vi "Aero_tunnel_monitor.vi"() -> ()   [LabVIEW 2010]
panel:
  out "ROAD SPEED_mps":dbl
  in  "BL Fan1":i32
  in  "BL Fan2":i32
  in  "Stop drive":bool
  in  "Start Drive":bool
  in  "Synch to Wind":bool
  out "Road Info":string
  in  "stop":bool
  out "Lift":dbl caption="N" format="%#.2f"
  out "Pitch":dbl caption="N.m" format="%#.2f"
  out "Drag":dbl caption="N" format="%#.2f"
  out "Side-Force":dbl caption="N" format="%#.2f"
  out "Yaw":dbl caption="N.m" format="%#.2f"
  out "Roll":dbl caption="N.m" format="%#.2f"
  out "SmAD Data":dbl[](array[numeric]) format="%.2f"
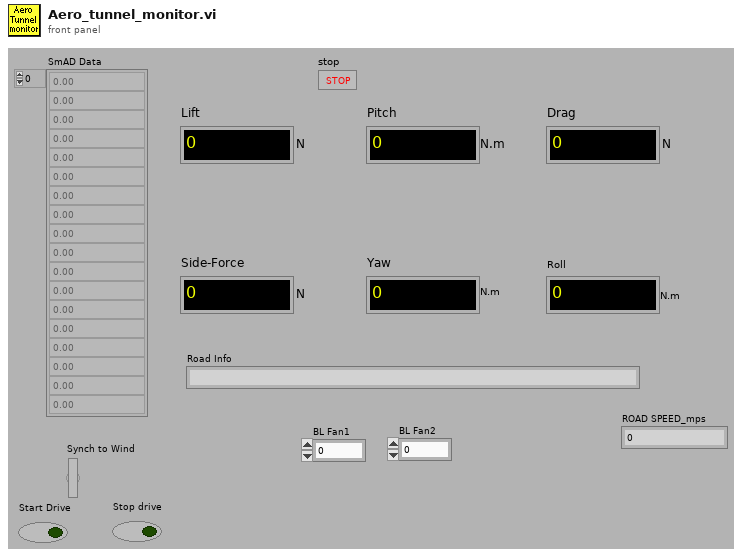
[diagram p1: front panel]
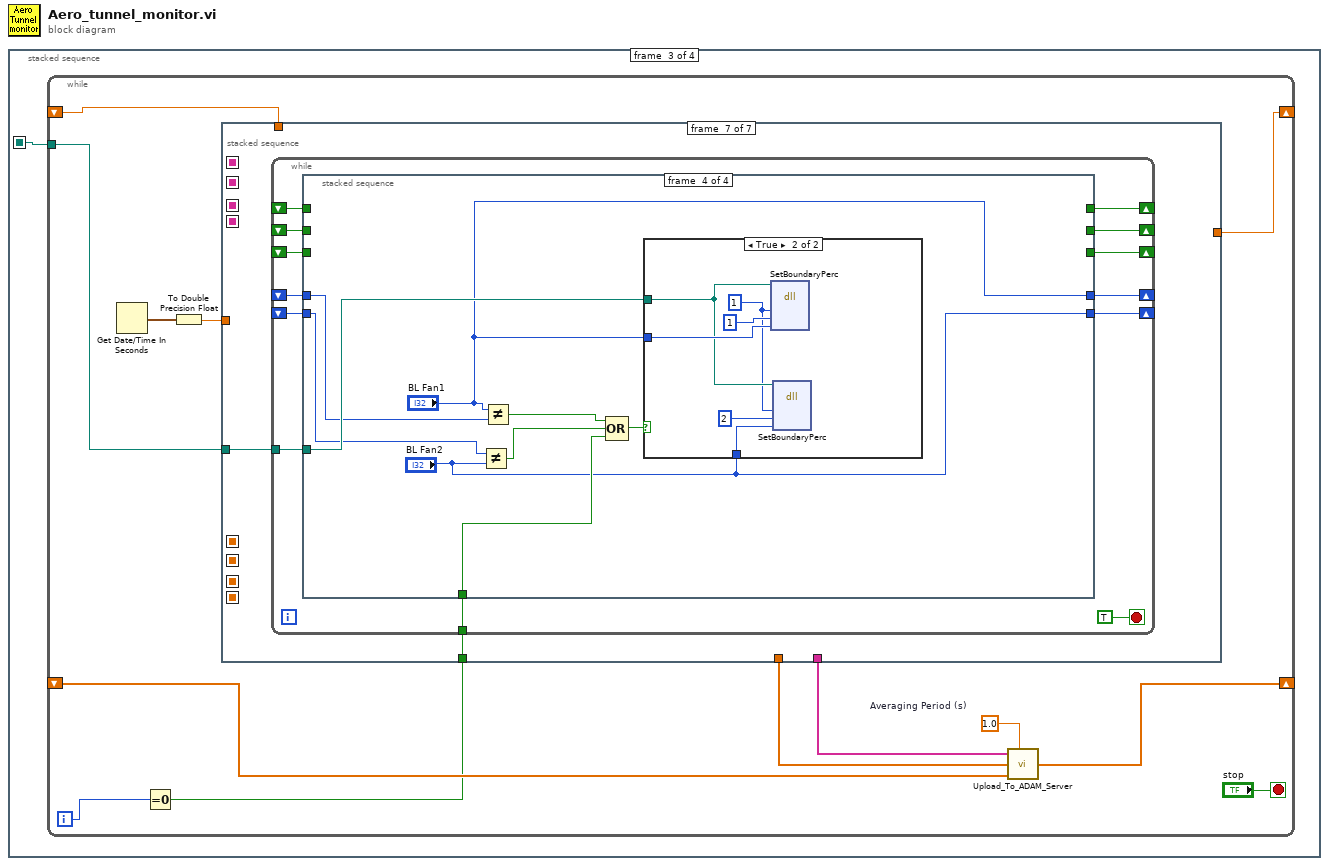
[diagram p0: block diagram]
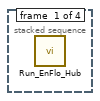
[diagram p2: hidden frame]
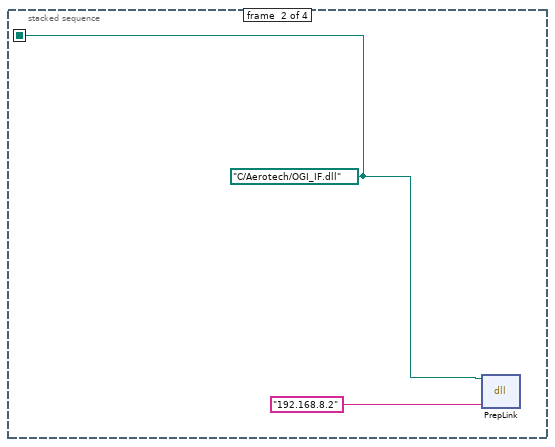
[diagram p3: hidden frame]
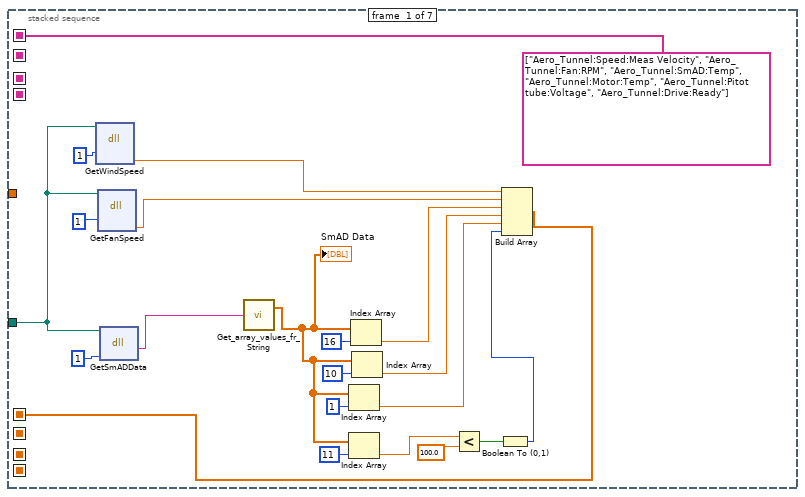
[diagram p4: hidden frame]
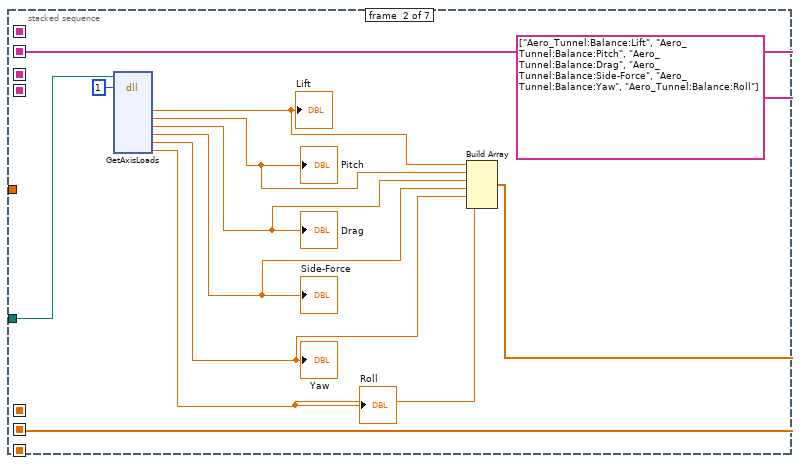
[diagram p5: hidden frame]
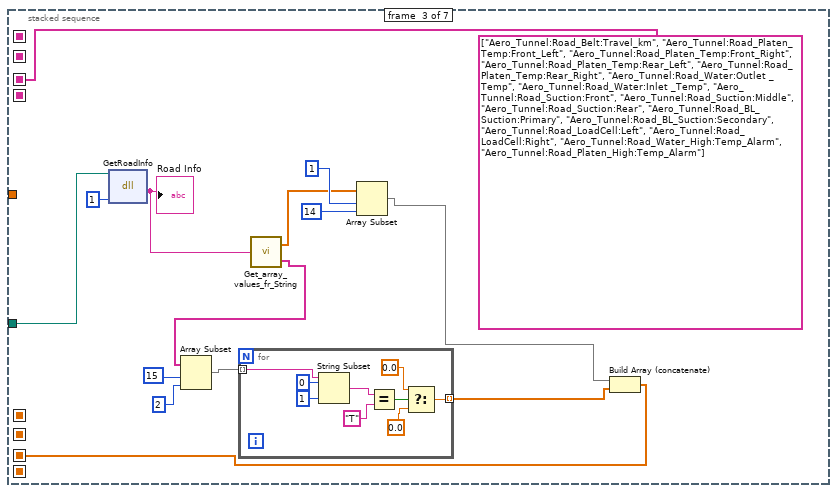
[diagram p6: hidden frame]
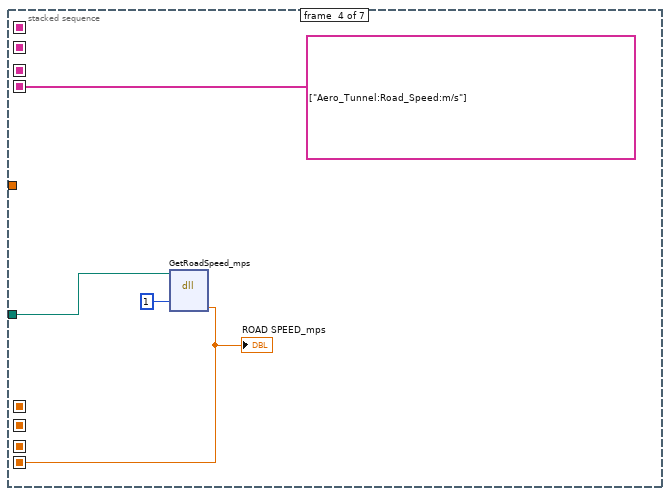
[diagram p7: hidden frame]
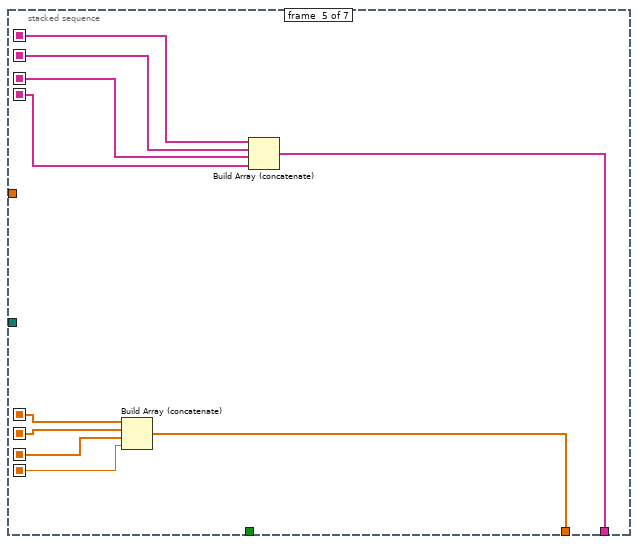
[diagram p8: hidden frame]
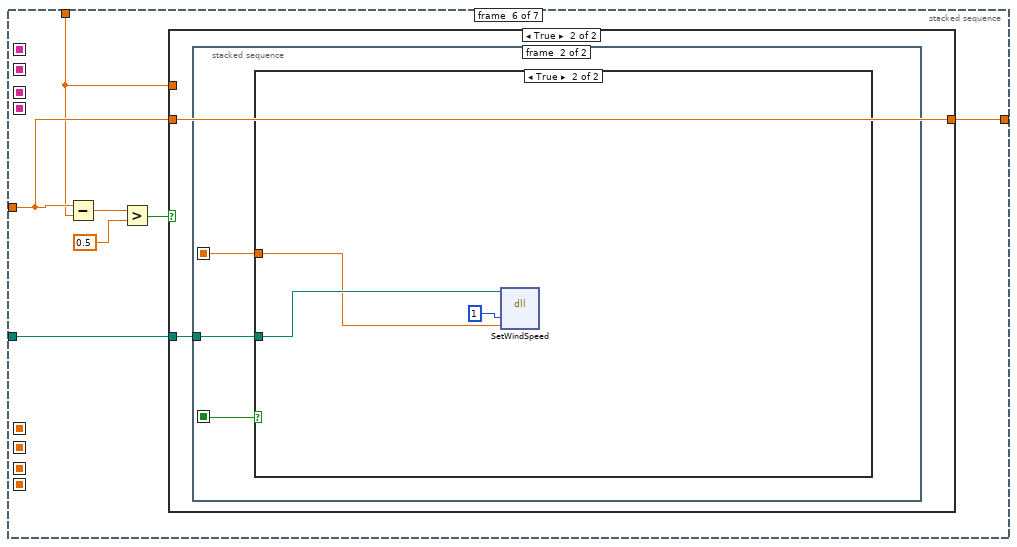
[diagram p9: hidden frame]
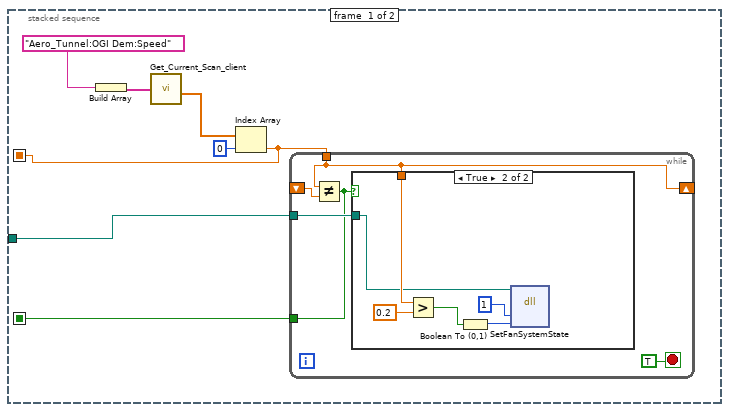
[diagram p11: hidden frame]
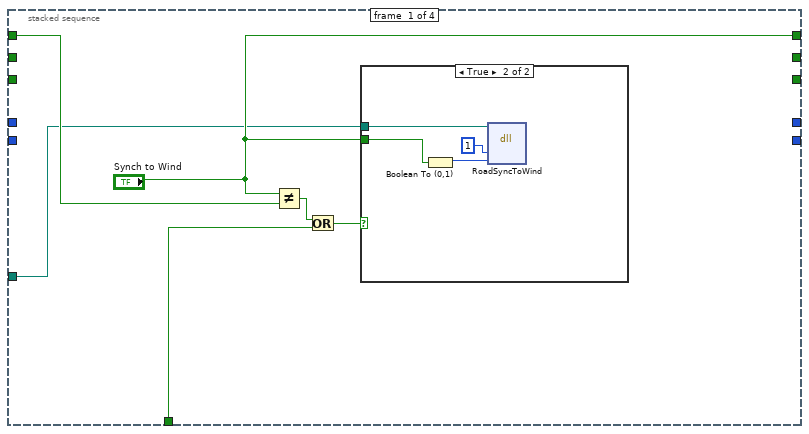
[diagram p14: hidden frame]
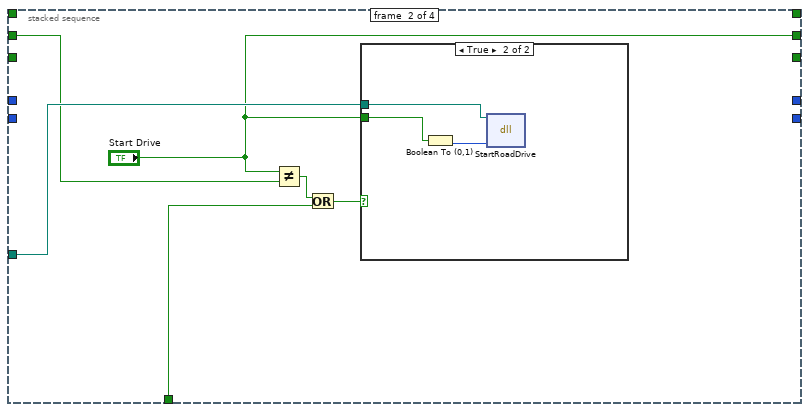
[diagram p16: hidden frame]
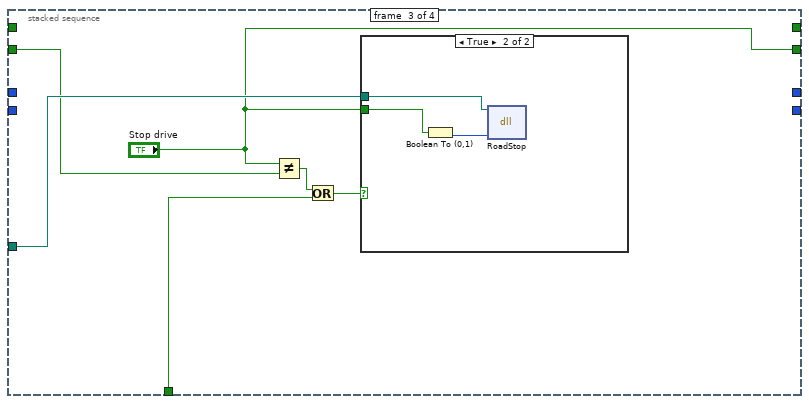
[diagram p18: hidden frame]
diagram:
  n1 = stacked-sequence {
    seq-local: [_ w1 _ _] -> [_ _ w3 w177]
    frame #0 {
      n2 = call "Run_EnFlo_Hub.vi"() -> ()  [unwired: 8 in]
    }
    frame #1 {
      w1 = path "C:/Aerotech/OGI_IF.dll" ("path in")
      n3 = dll-call lib="C:/Aerotech/Drivers/OGI_IF.dll" fn="PrepLink"(path in=w1, "IPAddress"="192.168.8.2") -> ()  [unwired: 2 in, 4 out]
    }
    frame #2 {
      n4 = while {
        shift-right: [w16] -> _
        shift-left: _ -> [w14]
        tunnel: w3 -> [w11]
        shift-right: [w6] -> _
        shift-left: _ -> [w9]
        i -> [w5]
        stop <- "stop" stop-if-true
        w12 = 1.0  # Averaging Period (s)
        n5 = Get Date/Time In Seconds() -> (seconds since 1Jan1904=w8:timestamp)
        n6 = Equal To 0?(x=w5) -> (x = 0?=w4:bool)
        n7 = To Double Precision Float(number=w8) -> (double precision float=w7:dbl)
        n8 = stacked-sequence {
          seq-local: [string[] ["Aero_Tunnel:Speed:Meas Velocity", "Aero_Tunnel:Fan:RPM", "Aero_Tunnel:SmAD:Temp", "Aero_Tunnel:Motor:Temp", "Aero_Tunnel:Pitot tube:Voltage", "Aero_Tunnel:Drive:Ready"] ("Channel Names") _ _ _ _ _ _] -> [_ _ _ _ w84 _ _]
          seq-local: [w25 _ _ _ _ _ _] -> [_ _ _ _ w82 _ _]
          seq-local: [_ string[] ["Aero_Tunnel:Balance:Lift", "Aero_Tunnel:Balance:Pitch", "Aero_Tunnel:Balance:Drag", "Aero_Tunnel:Balance:Side-Force", "Aero_Tunnel:Balance:Yaw", "Aero_Tunnel:Balance:Roll"] ("Channel Names") _ _ _ _ _] -> [_ _ _ _ w83 _ _]
          seq-local: [_ w46 _ _ _ _ _] -> [_ _ _ _ w81 _ _]
          seq-local: [_ _ w49 _ _ _ _] -> [_ _ _ _ w77 _ _]
          seq-local: [_ _ string[] ["Aero_Tunnel:Road_Belt:Travel_km", "Aero_Tunnel:Road_Platen_Temp:Front_Left", "Aero_Tunnel:Road_Platen_Temp:Front_Right", "Aero_Tunnel:Road_Platen_Temp:Rear_Left", "Aero_Tunnel:Road_Platen_Temp:Rear_Right", "Aero_Tunnel:Road_Water:Outlet _Temp", "Aero_Tunnel:Road_Water:Inlet _Temp", "Aero_Tunnel:Road_Suction:Front", "Aero_Tunnel:Road_Suction:Middle", "Aero_Tunnel:Road_Suction:Rear", "Aero_Tunnel:Road_BL_Suction:Primary", "Aero_Tunnel:Road_BL_Suction:Secondary", "Aero_Tunnel:Road_LoadCell:Left", "Aero_Tunnel:Road_LoadCell:Right", "Aero_Tunnel:Road_Water_High:Temp_Alarm", "Aero_Tunnel:Road_Platen_High:Temp_Alarm"] ("Channel Names") _ _ _ _] -> [_ _ _ _ w78 _ _]
          seq-local: [_ _ _ string[] ["Aero_Tunnel:Road_Speed:m/s"] ("Channel Names") _ _ _] -> [_ _ _ _ w76 _ _]
          seq-local: [_ _ _ w71 _ _ _] -> [_ _ _ _ w75 _ _]
          tunnel: [_ _ _ _ w80 _ _] -> w15
          tunnel: [_ _ _ _ w79 _ _] -> w13
          tunnel: w11 -> [w17 w44 w60 w73 _ w88 w119]
          tunnel: w7 -> [_ _ _ _ _ w86 _]
          tunnel: w9 -> [_ _ _ _ _ w85 _]
          tunnel: [_ _ _ _ _ w87 _] -> w6
          tunnel: w4 -> [_ _ _ _ _ _ w120]
          frame #0 {
            n9 = dll-call lib="C:/Aerotech/Drivers/OGI_IF.dll" fn="GetWindSpeed"(path in=w17, "Enable"=1) -> ("Windspeed_M/s"=w18:dbl)  [unwired: 3 in, 4 out]
            n10 = dll-call lib="C:/Aerotech/Drivers/OGI_IF.dll" fn="GetFanSpeed"(path in=w17, "Enable"=1) -> ("FanSpeedinRPM"=w19:dbl)  [unwired: 3 in, 4 out]
            n11 = dll-call lib="C:/Aerotech/Drivers/OGI_IF.dll" fn="GetSmADData"(path in=w17, "Enable"=1) -> ("SmAD Data String"=w22:string)  [unwired: 2 in, 3 out]
            n12 = call "Get_array_values_fr_String.vi"("String Value"=w22) -> ("Numeric Array"=w30:dbl[])  [unwired: 1 out]
            "SmAD Data" <- w30
            n13 = Index Array(array=w30, index=1) -> (element=w32:dbl)
            n14 = Index Array(array=w30, index=11) -> (element=w29:dbl)
            n15 = Index Array(array=w30, index=16) -> (element=w35:dbl)
            n16 = Index Array(array=w30, index=10) -> (element=w34:dbl)
            n17 = Less?(x=w29, y=100.0) -> (x < y?=w27:bool)
            n18 = Boolean To (0,1)(Boolean=w27) -> (0, 1=w26:i16)
            n19 = Build Array(w18, w19, w35, w34, w32, w26) -> (w25:dbl[])
          }
          frame #1 {
            n20 = dll-call lib="C:/Aerotech/Drivers/OGI_IF.dll" fn="GetAxisLoads"(path in=w44, "Enable"=1) -> ("Lift"=w43:dbl, "Pitch"=w42:dbl, "Drag"=w41:dbl, "side"=w40:dbl, "Yaw"=w39:dbl, "Roll"=w38:dbl)  [unwired: 3 in, 9 out]
            "Lift" <- w43
            "Pitch" <- w42
            "Drag" <- w41
            "Side-Force" <- w40
            "Yaw" <- w39
            "Roll" <- w38
            n21 = Build Array(w43, w42, w41, w40, w39, w38) -> (w46:dbl[])
          }
          frame #2 {
            n22 = dll-call lib="C:/Aerotech/Drivers/OGI_IF.dll" fn="GetRoadInfo"(path in=w60, "Enable"=1) -> ("Road Info"=w59:string)  [unwired: 3 in, 2 out]
            "Road Info" <- w59
            n23 = call "Get_array_values_fr_String.vi"("String Value"=w59) -> ("Numeric Array"=w56:dbl[], "String array"=w54:string[])
            n24 = Array Subset(array=w54, index=15, length=2) -> (w52:string[])
            n25 = for {
              tunnel: w52 -> [w68] mode=indexing
              tunnel: [w62] -> w51 mode=indexing
              n26 = String Subset(string=w68, offset (0)=0, length (rest)=1 ("length (rest)")) -> (substring=w67:string)
              n27 = Equal?(x=w67, y="T") -> (x = y?=w65:bool)
              n28 = Select(t=0.0, s=w65, f=0.0) -> (s? t:f=w62:dbl)
            }
            n29 = Array Subset(array=w56, index=1, length=14) -> (w50:dbl[])
            n30 = Build Array (concatenate)(w50, w51) -> (w49:dbl[])
          }
          frame #3 {
            n31 = dll-call lib="C:/Aerotech/Drivers/OGI_IF.dll" fn="GetRoadSpeed_mps"(path in=w73, "Enable"=1) -> ("RoadSpeed_mps"=w71:dbl)  [unwired: 3 in, 4 out]
            "ROAD SPEED_mps" <- w71
          }
          frame #4 {
            n32 = Build Array (concatenate)(w82, w81, w77, w75) -> (w80:dbl[])
            n33 = Build Array (concatenate)(w84, w83, w78, w76) -> (w79:string[])
          }
          frame #5 {
            n34 = Subtract(x=w86, y=w85) -> (x-y=w91:dbl)
            n35 = Greater?(x=w91, y=0.5) -> (0:w89:bool)
            n36 = case shown="True" w89 {
              tunnel: w88 -> [_ w94]
              tunnel: [w92 w93] -> w87
              tunnel: w86 -> [_ w93]
              tunnel: w85 -> [w92 _]
              frame False {
              }
              frame True {
                n37 = stacked-sequence {
                  seq-local: [w96 _] -> [_ w115]
                  seq-local: [w95 _] -> [_ w114]
                  tunnel: w94 -> [w99 w113]
                  frame #0 {
                    n38 = Build Array("Aero_Tunnel:OGI Dem:Speed") -> (w101:string[])
                    n39 = call "Get_Current_Scan_client.vi"("ADAM Ch Names"=w101) -> ("Numerical Values"=w98:dbl[])  [unwired: 1 in, 2 out]
                    n40 = Index Array(array=w98, index=0) -> (element=w96:dbl)
                    n41 = while {
                      tunnel: w99 -> [w106]
                      tunnel: w96 -> [w105]
                      shift-right: [w105] -> _
                      shift-left: _ -> [w104]
                      tunnel: [w102] -> w95
                      stop <- TRUE stop-if-true
                      n42 = Not Equal?(x=w105, y=w104) -> (x != y?=w102:bool)
                      n43 = case shown="True" w102 {
                        tunnel: w106 -> [_ w107]
                        tunnel: w105 -> [_ w108]
                        frame False {
                        }
                        frame True {
                          n44 = Greater?(x=w108, y=0.2) -> (0:w109:bool)
                          n45 = Boolean To (0,1)(Boolean=w109) -> (0, 1=w112:i16)
                          n46 = dll-call lib="C:/Aerotech/Drivers/OGI_IF.dll" fn="SetFanSystemState"(path in=w107, "Enable"=1, "Fan ONOFF"=w112) -> ()  [unwired: 3 in, 4 out]
                        }
                      }
                    }
                  }
                  frame #1 {
                    n47 = case shown="True" w114 {
                      tunnel: w115 -> [_ w117]
                      tunnel: w113 -> [_ w118]
                      frame False {
                      }
                      frame True {
                        n48 = dll-call lib="C:/Aerotech/Drivers/OGI_IF.dll" fn="SetWindSpeed"(path in=w118, "Enable"=1 ("t"), "NewWindSpeed"=w117) -> ()  [unwired: 4 in, 3 out]
                      }
                    }
                  }
                }
              }
            }
          }
          frame #6 {
            n49 = while {
              shift-right: [w131] -> _
              shift-left: _ -> [w133]
              tunnel: w120 -> [w132]
              tunnel: w119 -> [w129]
              shift-right: [w127] -> _
              shift-left: _ -> [w128]
              shift-right: [w125] -> _
              shift-left: _ -> [w126]
              shift-right: [w122] -> _
              shift-left: _ -> [w124]
              shift-right: [w121] -> _
              shift-left: _ -> [w123]
              stop <- TRUE stop-if-true
              n50 = stacked-sequence {
                tunnel: w133 -> [w139 _ _ _]
                tunnel: w132 -> [w137 w148 w157 w168]
                tunnel: ["Synch to Wind" _ _ _] -> w131
                tunnel: w129 -> [w134 w146 w155 w170]
                tunnel: w128 -> [_ w145 _ _]
                tunnel: [_ "Start Drive" _ _] -> w127
                tunnel: w126 -> [_ _ w154 _]
                tunnel: [_ _ "Stop drive" _] -> w125
                tunnel: w124 -> [_ _ _ w167]
                tunnel: w123 -> [_ _ _ w164]
                tunnel: [_ _ _ "BL Fan1"] -> w122
                tunnel: [_ _ _ "BL Fan2"] -> w121
                frame #0 {
                  n51 = Not Equal?(x="Synch to Wind", y=w139) -> (x != y?=w138:bool)
                  n52 = Or(x=w138, y=w137) -> (x .or. y?=w135:bool)
                  n53 = case shown="True" w135 {
                    tunnel: "Synch to Wind" -> [_ w141]
                    tunnel: w134 -> [_ w140]
                    frame False {
                    }
                    frame True {
                      n54 = Boolean To (0,1)(Boolean=w141) -> (0, 1=w142:i16)
                      n55 = dll-call lib="C:/Aerotech/Drivers/OGI_IF.dll" fn="RoadSyncToWind"(path in=w140, "Enable"=1, "SynchState"=w142) -> ()  [unwired: 3 in, 4 out]
                    }
                  }
                }
                frame #1 {
                  n56 = Not Equal?(x="Start Drive", y=w145) -> (x != y?=w149:bool)
                  n57 = Or(x=w149, y=w148) -> (x .or. y?=w147:bool)
                  n58 = case shown="True" w147 {
                    tunnel: "Start Drive" -> [_ w152]
                    tunnel: w146 -> [_ w150]
                    frame False {
                    }
                    frame True {
                      n59 = Boolean To (0,1)(Boolean=w152) -> (0, 1=w151:i16)
                      n60 = dll-call lib="C:/Aerotech/Drivers/OGI_IF.dll" fn="StartRoadDrive"(path in=w150, "Enable"=w151) -> ()  [unwired: 2 in, 4 out]
                    }
                  }
                }
                frame #2 {
                  n61 = Not Equal?(x="Stop drive", y=w154) -> (x != y?=w158:bool)
                  n62 = Or(x=w158, y=w157) -> (x .or. y?=w156:bool)
                  n63 = case shown="True" w156 {
                    tunnel: "Stop drive" -> [_ w161]
                    tunnel: w155 -> [_ w159]
                    frame False {
                    }
                    frame True {
                      n64 = Boolean To (0,1)(Boolean=w161) -> (0, 1=w160:i16)
                      n65 = dll-call lib="C:/Aerotech/Drivers/OGI_IF.dll" fn="RoadStop"(path in=w159, "Enable"=w160) -> ()  [unwired: 2 in, 4 out]
                    }
                  }
                }
                frame #3 {
                  n66 = Not Equal?(x=w164, y="BL Fan2") -> (x != y?=w165:bool)
                  n67 = Not Equal?(x="BL Fan1", y=w167) -> (x != y?=w166:bool)
                  n68 = Compound Arithmetic op=OR(w166, w165, w168) -> (w169:bool)
                  n69 = case shown="True" w169 {
                    tunnel: w170 -> [_ w172]
                    tunnel: "BL Fan1" -> [_ w174]
                    tunnel: "BL Fan2" -> [_ w173]
                    frame False {
                    }
                    frame True {
                      w171 = 1 ("BL Fan (1 or 2)")
                      n70 = dll-call lib="C:/Aerotech/Drivers/OGI_IF.dll" fn="SetBoundaryPerc"(path in=w172, "enable"=w171, "BL Fan (1 or 2)"=1, "New Percentage"=w174) -> ()  [unwired: 4 in, 4 out]
                      n71 = dll-call lib="C:/Aerotech/Drivers/OGI_IF.dll" fn="SetBoundaryPerc"(path in=w172, "enable"=w171, "BL Fan (1 or 2)"=2, "New Percentage"=w173) -> ()  [unwired: 4 in, 4 out]
                    }
                  }
                }
              }
            }
          }
        }
        n72 = call "Upload_To_ADAM_Server.vi"("Channel Names"=w13, "Averaging Period (s)"=w12, "Channel Values"=w15, "Shift In"=w14) -> ("Shift Out"=w16:dbl[])  [unwired: 1 out]
      }
    }
    frame #3 {
      n73 = dll-call lib="C:/Aerotech/Drivers/OGI_IF.dll" fn="CloseLink"(path in=w177) -> ()  [unwired: 2 in, 3 out]
    }
  }
